vi "orderbook.test.Reduce.Size.vi"(8 "error in":errorcluster) -> (0 "error out":errorcluster, 3 "Passed":bool)   [LabVIEW 2020]
uses:
  arty/orderbook/orderbook.command.ctl
  arty/orderbook/orderbook.command.type.ctl
  arty/application/orderbook.entry.ctl
  arty/application/orderbook.result.type.ctl
panel:
  out "output cluster":T1
  out "OrderBook.Entries":T2[](array[typedef]) {"Side (U8)" format="%.0x"}
  in  "OrderBook.Command[]\nto Send":T4[](array[typedef])=[{"OrderBook Command.Type"=enum."AddOrder", "Side (U8)"=66, "Order Id (U64)"=336, "Quantity (U32)"=130, "Symbol (U64)"=29033, "Price (U64)"=9525, "Executed Quantity (U32)"=0, "Cancelled Quantity (U32)"=0}, {"OrderBook Command.Type"=enum."AddOrder", "Side (U8)"=66, "Order Id (U64)"=337, "Quantity (U32)"=225, "Symbol (U64)"=29033, "Price (U64)"=9115, "Executed Quantity (U32)"=0, "Cancelled Quantity (U32)"=0}, {"OrderBook Command.Type"=enum."ReduceSize", "Side (U8)"=66, "Order Id (U64)"=336, "Quantity (U32)"=0, "Symbol (U64)"=29033, "Price (U64)"=9200, "Executed Quantity (U32)"=0, "Cancelled Quantity (U32)"=0}, {"OrderBook Command.Type"=enum."Get.Top", "Side (U8)"=0, "Order Id (U64)"=0, "Quantity (U32)"=0, "Symbol (U64)"=0, "Price (U64)"=0, "Executed Quantity (U32)"=0, "Cancelled Quantity (U32)"=0}] {"Side (U8)" format="%.0x"; "Order Id (U64)" format="%.0x"; "Symbol (U64)" format="%.0x"}
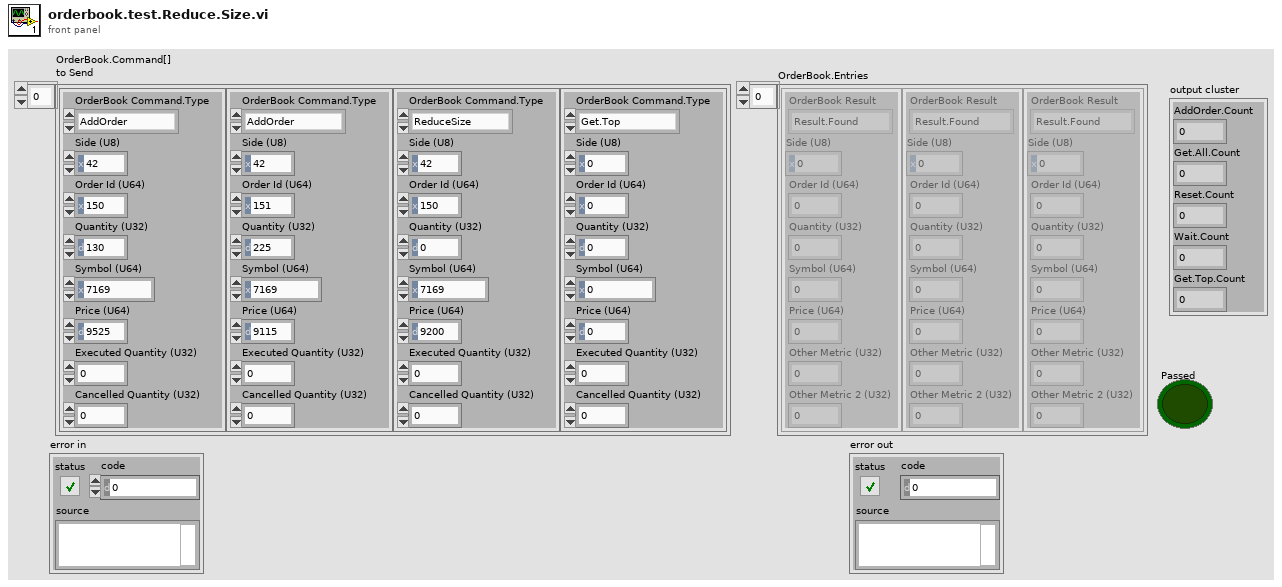
[diagram p1: front panel]
types:
  T1 = cluster{"AddOrder.Count":u32, "Get.All.Count":u32, "Reset.Count":u32, "Wait.Count":u32, "Get.Top.Count":u32}
  T2 = typedef "orderbook.entry.ctl" = cluster{"OrderBook Result":T3, "Side (U8)":u8, "Order Id (U64)":u64, "Quantity (U32)":u32, "Symbol (U64)":u64, "Price (U64)":u64, "Other Metric (U32)":u32, "Other Metric 2 (U32)":u32}
  T3 = typedef "orderbook.result.type.ctl" = enum16{"Result.Found", "Result.Not.Found"}
  T4 = typedef "orderbook.command.ctl" = cluster{"OrderBook Command.Type":T5, "Side (U8)":u8, "Order Id (U64)":u64, "Quantity (U32)":u32, "Symbol (U64)":u64, "Price (U64)":u64, "Executed Quantity (U32)":u32, "Cancelled Quantity (U32)":u32}
  T5 = typedef "orderbook.command.type.ctl" = enum16{"AddOrder", "OrderExecuted", "ReduceSize", "ModifyOrder", "DeleteOrder", "Get.All.Orders", "Get.Top"}
  T6 = cluster{"Write.Request":bool, "Read.Request":bool, "Read.Address":u32, "Read.OrderBook.Entry":cluster{"OrderBook Result":enum16{"Result.Found", "Result.Not.Found"}, "Side (U8)":u8, "Order Id (U64)":u64, "Quantity (U32)":u32, "Symbol (U64)":u64, "Price (U64)":u64, "Other Metric (U32)":u32, "Other Metric 2 (U32)":u32}, "Number.of.Entries":u32, "OrderBook.State":enum16{"Reset", "WaitForNewCommand", "AddOrder", "Get.All.Orders", "Get.Top"}, "Ready.For.OrderBook.Command":bool, "Memory.State":enum16{"New", "Request.Data", "Append", "Data.Ready"}, "Move":bool, "Read.Valid":bool, "Write.Address":u32, "Write.OrderBook.Entry":cluster{"OrderBook Result":enum16{"Result.Found", "Result.Not.Found"}, "Side (U8)":u8, "Order Id (U64)":u64, "Quantity (U32)":u32, "Symbol (U64)":u64, "Price (U64)":u64, "Other Metric (U32)":u32, "Other Metric 2 (U32)":u32}, "OrderBook.Result.Valid":bool, "AddOrder.Count":u32, "Get.All.Count":u32, "Reset.Count":u32, "Wait.Count":u32, "Append":bool, "Get.Top.Count":u32}
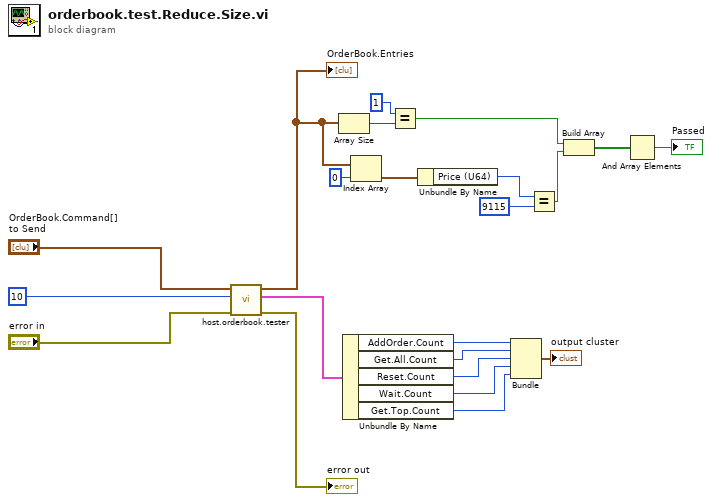
[diagram p0: block diagram]
diagram:
  n1 = call "host.orderbook.tester.vi"("error in"="error in", "Seconds to Wait"=10 ("Seconds\nto\nWait"), "OrderBook.Command[]\nto Send"="OrderBook.Command[]\nto Send") -> ("error out"=→"error out":errorcluster, "OrderBook.Variables"=w6:T6, "OrderBook.Entries"=w4:T2[])  [unwired: 6 in]
  "OrderBook.Entries" <- w4
  n2 = Array Size(array=w4) -> (size(s)=w15:i32)
  n3 = Unbundle By Name(w6) -> ("AddOrder.Count"=w19:u32, "Get.All.Count"=w16:u32, "Reset.Count"=w17:u32, "Wait.Count"=w18:u32, "Get.Top.Count"=w2:u32)
  n4 = Index Array(array=w4, index=0) -> (element=w13:T2)
  n5 = Equal?(x=1, y=w15) -> (x = y?=w9:bool)
  n6 = Unbundle By Name(w13) -> ("Price (U64)"=w11:u64)
  n7 = Bundle("AddOrder.Count"=w19, "Get.All.Count"=w16, "Reset.Count"=w17, "Wait.Count"=w18, "Get.Top.Count"=w2) -> (→"output cluster":T1)  [unwired: 1 in]
  n8 = Equal?(x=w11, y=u64 9115) -> (x = y?=w10:bool)
  n9 = Build Array(w9, w10) -> (w8:bool[])
  n10 = And Array Elements(Boolean array=w8) -> (logical AND=→"Passed":bool)
